vi "To Variant.vi"(8 "error in (no error)":errorcluster, 9 "datatype and defaults":variant, 11 "JSON Value in":refnum<class "JSON Value.lvclass">) -> (0 "error out":errorcluster, 1 "defaulted keys":string[](array[string]), 2 "Variant":variant)   [LabVIEW 2016, in "JSON Value.lvclass"]
doc: "Populates a variant with the data contained in the given JSON instance. Valid types for datatype and defaults are: string, boolean, double, and a cluster of named controls of strings, booleans, doubles, or nested clusters.\n\nIf a given cluster contains values that aren't present in the JSON Object instance, the value in the datatype and defaults control is used instead and the defaulted keys output will contain the name of the path in the cluster to the control."
uses:
  JSON Value.lvclass
  JSON Types.ctl
  JSON String/Read value as String.vi
  <vilib>/Utility/Data Type/NI_Data Type.lvlib
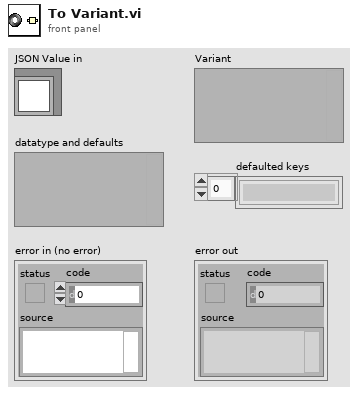
[diagram p1: front panel]
types:
  T1 = typedef "JSON Value.lvclass/JSON Types.ctl" = enum16{"String", "Numeric", "Boolean", "NULL", "Object", "Array"}
  T2 = typedef "NI_Data Type.lvlib/Data Type.ctl" = enum8{"Invalid Type", "Void", "I8", "I16", "I32", "I64", "U8", "U16", "U32", "U64", "Single Float", "Double Float", "Extended Float", "Single Complex", "Double Complex", "Extended Complex", "Enum U8", "Enum U16", "Enum U32", "Enum U64", "Single Float With Unit", "Double Float With Unit", "Extended Float With Unit", "Single Complex with Unit", "Double Complex with Unit", "Extended Complex with Unit", "Boolean", "String", "Path", "Picture", "Tag", "Array", "Cluster", "Variant", "LV Variant", "Waveform", "Timestamp", "Digital Waveform", "Digital Data", "ExpressData", "Refnum", "External Data", "VI", "Poly VI", "LabVIEW Class Instance", "Fixed Point"}
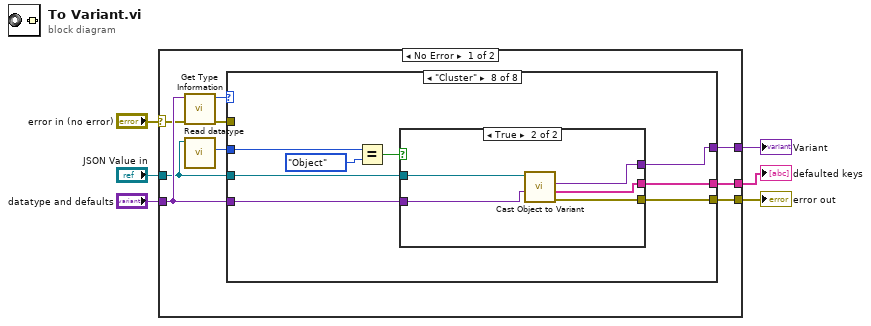
[diagram p0: block diagram]
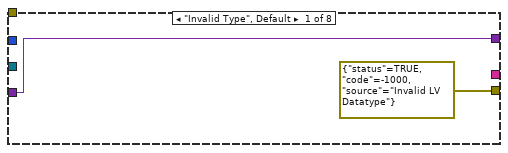
[diagram p2: hidden frame]
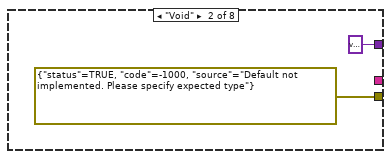
[diagram p3: hidden frame]
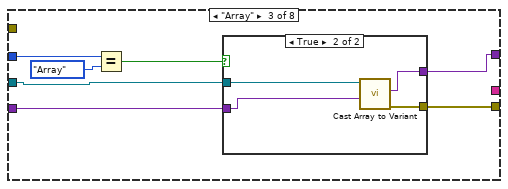
[diagram p4: hidden frame]
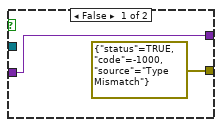
[diagram p5: hidden frame]
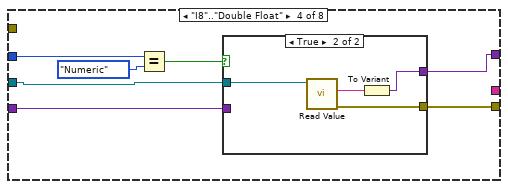
[diagram p6: hidden frame]
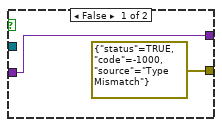
[diagram p7: hidden frame]
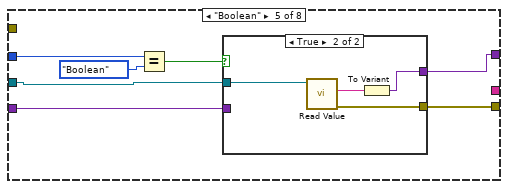
[diagram p8: hidden frame]
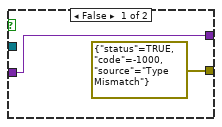
[diagram p9: hidden frame]
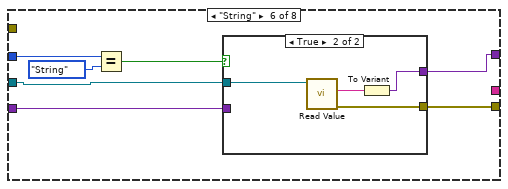
[diagram p10: hidden frame]
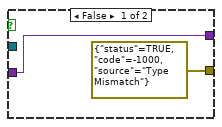
[diagram p11: hidden frame]
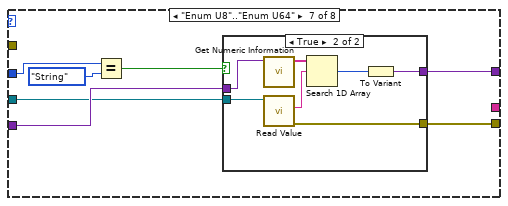
[diagram p12: hidden frame]
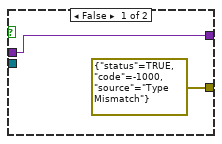
[diagram p13: hidden frame]
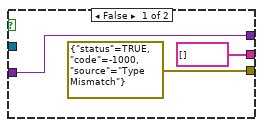
[diagram p14: hidden frame]
diagram:
  n1 = case shown="No Error" "error in (no error)" {
    selector: "error in (no error)" -> [w12 w105]
    tunnel: [w10 w105] -> w5
    tunnel: "JSON Value in" -> [w8 _]
    tunnel: "datatype and defaults" -> [w13 w104]
    tunnel: [w14 w104] -> w2
    tunnel: [w9 _] -> w1
    frame No Error {
      n2 = call <vilib>:"Get Type Information.vi"("error in (no error)"=w12, "Variant"=w13) -> ("error out"=w11:errorcluster, "Type"=w15:T2)  [unwired: 5 in, 3 out]
      n3 = call "Read datatype.vi"("JSON Value in"=w8) -> ("datatype"=w7:T1)  [unwired: 8 in, 2 out]
      n4 = case shown="\"Cluster\"" w15 {
        tunnel: w8 -> [_ _ w23 w34 w49 w62 w75 w91]
        tunnel: [w17 variant ("datatype and defaults") w24 w37 w51 w64 w77 w94] -> w14
        tunnel: w13 -> [w17 _ w25 w39 w52 w63 w76 w95]
        tunnel: w11 -> [_ _ _ _ _ _ _ _]
        tunnel: [errorcluster {"status"=TRUE, "code"=-1000, "source"="Invalid LV Datatype"} ("error out") errorcluster {"status"=TRUE, "code"=-1000, "source"="Default not implemented. Please specify expected type"} ("error out") w26 w38 w50 w65 w78 w93] -> w10
        tunnel: [_ _ _ _ _ _ _ w92] -> w9
        tunnel: w7 -> [_ _ w22 w36 w48 w61 w74 w90]
        frame "Invalid Type", Default {
        }
        frame "Void" {
        }
        frame "Array" {
          n5 = Equal?(x=w22, y=JSON_Types."Array") -> (x = y?=w20:bool)
          n6 = case shown="True" w20 {
            tunnel: [errorcluster {"status"=TRUE, "code"=-1000, "source"="Type Mismatch"} ("error out") w31] -> w26
            tunnel: [w28 w32] -> w24
            tunnel: w25 -> [w28 w29]
            tunnel: w23 -> [_ w30]
            frame False {
            }
            frame True {
              n7 = call "Cast Array to Variant.vi"("datatype and defaults"=w29, "JSON Value in"=w30) -> ("error out"=w31:errorcluster, "Variant"=w32:variant)  [unwired: 8 in]
            }
          }
        }
        frame "I8".."Double Float" {
          n8 = Equal?(x=w36, y=JSON_Types."Numeric") -> (x = y?=w33:bool)
          n9 = case shown="True" w33 {
            tunnel: w34 -> [_ w45]
            tunnel: [errorcluster {"status"=TRUE, "code"=-1000, "source"="Type Mismatch"} ("error out") w44] -> w38
            tunnel: [w41 w43] -> w37
            tunnel: w39 -> [w41 _]
            frame False {
            }
            frame True {
              n10 = call-poly "Read Value.vi"("JSON Value in"=w45) -> ("error out"=w44:errorcluster, "value"=w42:string)  [unwired: 9 in]
              n11 = To Variant(anything=w42) -> (Variant=w43:variant)
            }
          }
        }
        frame "Boolean" {
          n12 = Equal?(x=w48, y=JSON_Types."Boolean") -> (x = y?=w46:bool)
          n13 = case shown="True" w46 {
            tunnel: w49 -> [_ w58]
            tunnel: [errorcluster {"status"=TRUE, "code"=-1000, "source"="Type Mismatch"} ("error out") w57] -> w50
            tunnel: [w54 w56] -> w51
            tunnel: w52 -> [w54 _]
            frame False {
            }
            frame True {
              n14 = call-poly "Read Value.vi"("JSON Value in"=w58) -> ("error out"=w57:errorcluster, "value"=w55:string)  [unwired: 9 in]
              n15 = To Variant(anything=w55) -> (Variant=w56:variant)
            }
          }
        }
        frame "String" {
          n16 = Equal?(x=w61, y=JSON_Types."String") -> (x = y?=w59:bool)
          n17 = case shown="True" w59 {
            tunnel: w62 -> [_ w71]
            tunnel: [errorcluster {"status"=TRUE, "code"=-1000, "source"="Type Mismatch"} ("error out") w70] -> w65
            tunnel: [w67 w69] -> w64
            tunnel: w63 -> [w67 _]
            frame False {
            }
            frame True {
              n18 = call-poly "Read Value.vi"("JSON Value in"=w71) -> ("error out"=w70:errorcluster, "value"=w68:string)  [unwired: 9 in]
              n19 = To Variant(anything=w68) -> (Variant=w69:variant)
            }
          }
        }
        frame "Enum U8".."Enum U64" {
          n20 = Equal?(x=w74, y=JSON_Types."String") -> (x = y?=w72:bool)
          n21 = case shown="True" w72 {
            tunnel: [errorcluster {"status"=TRUE, "code"=-1000, "source"="Type Mismatch"} ("error out") w87] -> w78
            tunnel: [w80 w86] -> w77
            tunnel: w76 -> [w80 w85]
            tunnel: w75 -> [_ w81]
            frame False {
            }
            frame True {
              n22 = call <vilib>:"Get Numeric Information.vi"("Variant"=w85) -> ("Enum Names"=w83:string[])  [unwired: 7 in, 3 out]
              n23 = call-poly "Read Value.vi"("JSON Value in"=w81) -> ("error out"=w87:errorcluster, "value"=w84:string)  [unwired: 9 in]
              n24 = Search 1D Array(1D array=w83, element=w84) -> (index of element=w82:i32)  [unwired: 1 in]
              n25 = To Variant(anything=w82) -> (Variant=w86:variant)
            }
          }
        }
        frame "Cluster" {
          n26 = Equal?(x=w90, y=JSON_Types."Object") -> (x = y?=w88:bool)
          n27 = case shown="True" w88 {
            tunnel: w95 -> [w98 w103]
            tunnel: [w98 w102] -> w94
            tunnel: [errorcluster {"status"=TRUE, "code"=-1000, "source"="Type Mismatch"} ("error out") w101] -> w93
            tunnel: [string[] [] ("defaulted keys") w100] -> w92
            tunnel: w91 -> [_ w99]
            frame False {
            }
            frame True {
              n28 = call "Cast Object to Variant.vi"("datatype and defaults"=w103, "JSON Value in"=w99) -> ("error out"=w101:errorcluster, "defaulted keys"=w100:string[], "Variant"=w102:variant)  [unwired: 7 in]
            }
          }
        }
      }
    }
    frame Error {
    }
  }
  "error out" <- w5
  "Variant" <- w2
  "defaulted keys" <- w1
